vi "StepAmplitude.vi"() -> ()   [LabVIEW 2013]
uses:
  C:/Code/Apps/Utilities/AG-UC2-UC8/AG-UC2-UC8/Install/Samples/LabVIEW/LabVIEW 2013/CmdLibAgilis.dll
  CmdLibAgilis.dll
panel:
  out "Output:":string
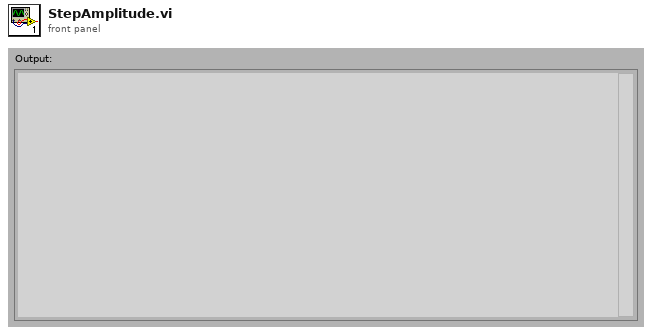
[diagram p1: front panel]
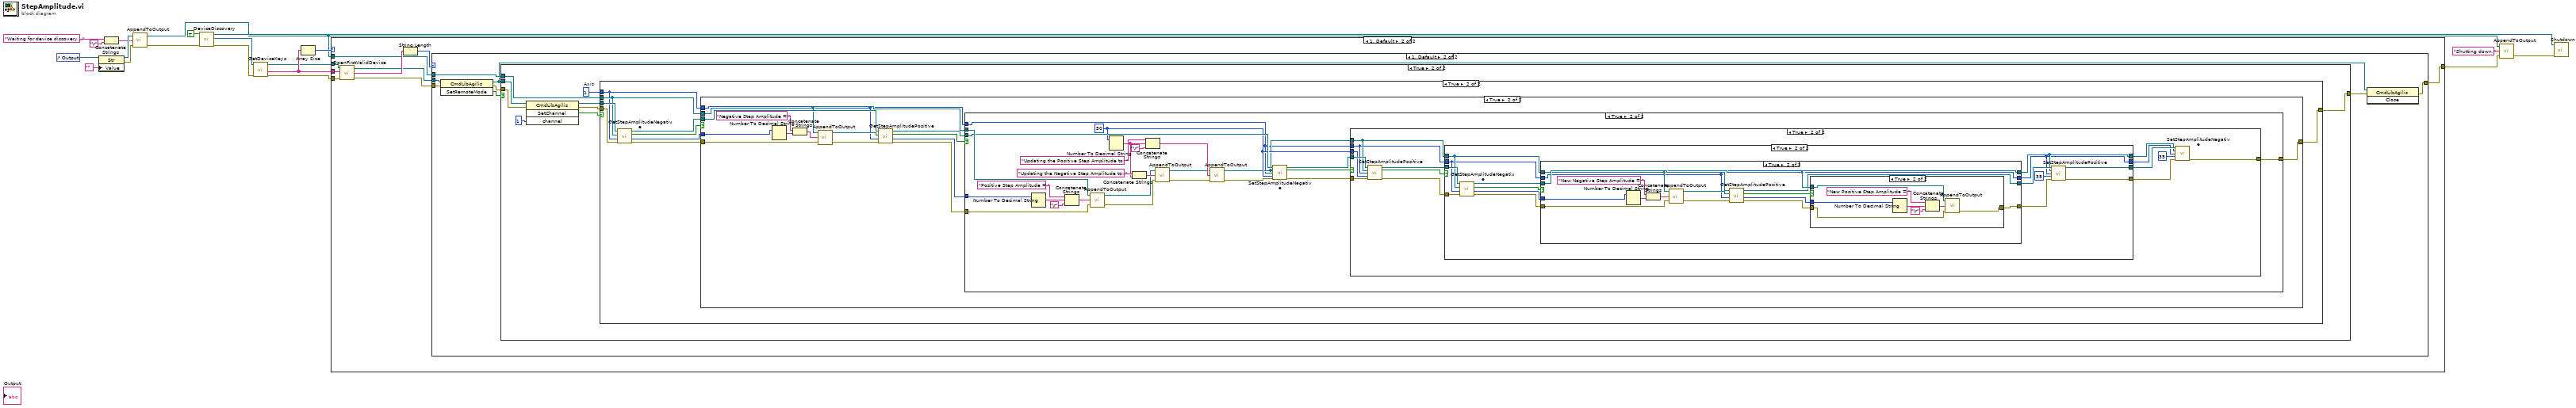
[diagram p0: block diagram]
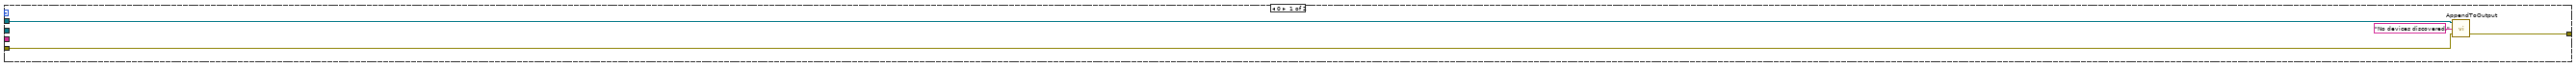
[diagram p2: hidden frame]
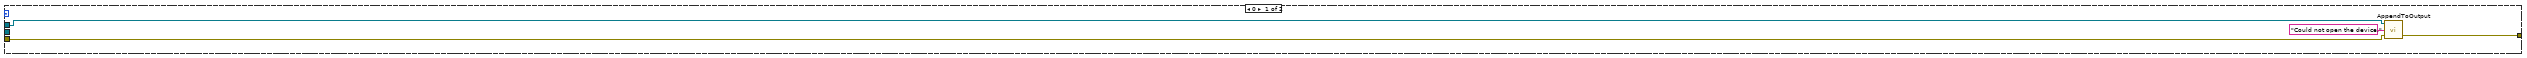
[diagram p3: hidden frame]
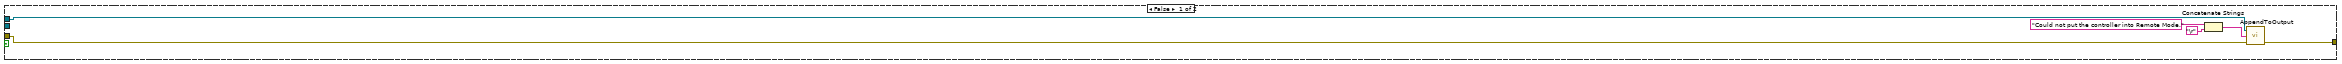
[diagram p4: hidden frame]
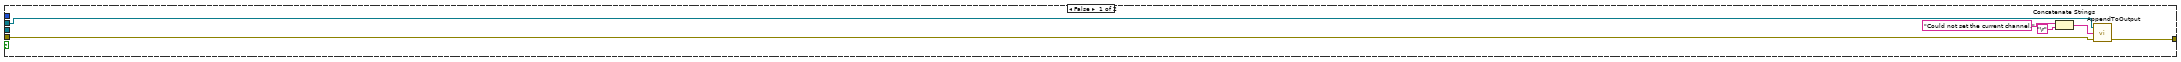
[diagram p5: hidden frame]
diagram:
  n1 = control-ref of="Output:"() -> (w20:refnum<vi>)
  n2 = property class="Str"(reference=w20, "Value"="") -> (reference out=w17:refnum<vi>, error out=w18:errorcluster)  [unwired: 1 in]
  n3 = Concatenate Strings("Waiting for device discovery...", "\r") -> (w7:string)
  n4 = call "AppendToOutput.vi"("error in"=w18, "Input String"=w7, "Output Refnum In"=w17) -> ("error out"=w15:errorcluster, "Output Refnum Out"=w1:refnum<vi>)  [unwired: 1 in]
  n5 = call "DeviceDiscovery.vi"("error in (no error)"=w15, "logging"=TRUE) -> ("error out"=w14:errorcluster, "CmdLib Out"=w13:refnum<k24>, "VCPIOLib Out"=w10:refnum<k24>)  [unwired: 3 in]
  n6 = call "GetDeviceKeys.vi"("error in (no error)"=w14, "CmdLib In"=w13) -> ("error out"=w11:errorcluster, "Device Keys"=w9:string[], "CmdLib Out"=w8:refnum<k24>)  [unwired: 3 in]
  n7 = Array Size(array=w9) -> (size(s)=w12:i32)
  n8 = case shown="1, Default" w12 {
    tunnel: w1 -> [w24 w28]
    tunnel: w11 -> [w23 w32]
    tunnel: w9 -> [_ w31]
    tunnel: w8 -> [_ w33]
    tunnel: [w21 w25] -> w2
    frame 0 {
      n9 = call "AppendToOutput.vi"("error in"=w23, "Input String"="No devices discovered.", "Output Refnum In"=w24) -> ("error out"=w21:errorcluster)  [unwired: 1 in, 1 out]
    }
    frame 1, Default {
      n10 = call "OpenFirstValidDevice.vi"("error in (no error)"=w32, "Device Keys"=w31, "CmdLib In"=w33) -> ("error out"=w27:errorcluster, "DeviceKey Out"=w30:string, "CmdLib Out"=w26:refnum<k24>)  [unwired: 1 in]
      n11 = String Length(string=w30) -> (length=w29:i32)
      n12 = case shown="1, Default" w29 {
        tunnel: w28 -> [w36 w42]
        tunnel: w27 -> [w35 w45]
        tunnel: w26 -> [_ w44]
        tunnel: [w34 w39] -> w25
        frame 0 {
          n13 = call "AppendToOutput.vi"("error in"=w35, "Input String"="Could not open the device." ("DeviceKey Out"), "Output Refnum In"=w36) -> ("error out"=w34:errorcluster)  [unwired: 1 in, 1 out]
        }
        frame 1, Default {
          n14 = invoke class="CmdLibAgilis" method="SetRemoteMode"(reference=w44, error in=w45) -> (reference out=w38:refnum<k24>, error out=w43:errorcluster, "SetRemoteMode"=w41:bool)  [unwired: 1 in]
          n15 = case shown="True" w41 {
            tunnel: w43 -> [w51 w60]
            tunnel: w42 -> [w47 w55]
            tunnel: w38 -> [_ w59]
            tunnel: [w46 w54] -> w40
            frame False {
              n16 = Concatenate Strings("Could not put the controller into Remote Mode." ("DeviceKey Out"), "\r") -> (w50:string)
              n17 = call "AppendToOutput.vi"("error in"=w51, "Input String"=w50, "Output Refnum In"=w47) -> ("error out"=w46:errorcluster)  [unwired: 1 in, 1 out]
            }
            frame True {
              w52 = 1  # Axis
              n18 = invoke class="CmdLibAgilis" method="SetChannel"(reference=w59, error in=w60, "channel"=1) -> (reference out=w53:refnum<k24>, error out=w56:errorcluster, "SetChannel"=w57:bool)  [unwired: 1 in, 1 out]
              n19 = case shown="True" w57 {
                tunnel: w55 -> [w66 w70]
                tunnel: w56 -> [w65 w74]
                tunnel: [w61 w71] -> w54
                tunnel: w53 -> [_ w75]
                tunnel: w52 -> [_ w68]
                frame False {
                  n20 = Concatenate Strings("Could not set the current channel." ("DeviceKey Out"), "\r") -> (w64:string)
                  n21 = call "AppendToOutput.vi"("error in"=w65, "Input String"=w64, "Output Refnum In"=w66) -> ("error out"=w61:errorcluster)  [unwired: 1 in, 1 out]
                }
                frame True {
                  n22 = call "GetStepAmplitudeNegative.vi"("error in (no error)"=w74, "Axis"=w68, "Output Refnum In"=w70, "CmdLib In"=w75) -> ("error out"=w69:errorcluster, "Step Amplitude"=w73:i32, "GetStepAmplitudeNegative"=w72:bool, "CmdLib Out"=w67:refnum<k24>)  [unwired: 4 in]
                  n23 = case shown="True" w72 {
                    tunnel: w73 -> [_ w90]
                    tunnel: [w76 w79] -> w71
                    tunnel: w70 -> [_ w80]
                    tunnel: w69 -> [w76 w87]
                    tunnel: w68 -> [_ w78]
                    tunnel: w67 -> [_ w84]
                    frame False {
                    }
                    frame True {
                      n24 = Number To Decimal String(number=w90) -> (decimal integer string=w89:string)  [unwired: 1 in]
                      n25 = Concatenate Strings("Negative Step Amplitude = ", w89) -> (w88:string)
                      n26 = call "AppendToOutput.vi"("error in"=w87, "Input String"=w88, "Output Refnum In"=w80) -> ("error out"=w86:errorcluster, "Output Refnum Out"=w85:refnum<vi>)  [unwired: 1 in]
                      n27 = call "GetStepAmplitudePositive.vi"("error in (no error)"=w86, "Axis"=w78, "Output Refnum In"=w85, "CmdLib In"=w84) -> ("error out"=w81:errorcluster, "Step Amplitude"=w82:i32, "GetStepAmplitudePositive"=w83:bool, "CmdLib Out"=w77:refnum<k24>)  [unwired: 4 in]
                      n28 = case shown="True" w83 {
                        tunnel: w82 -> [_ w115]
                        tunnel: w81 -> [w92 w114]
                        tunnel: w80 -> [_ w113]
                        tunnel: [w92 w93] -> w79
                        tunnel: w78 -> [_ w94]
                        tunnel: w77 -> [_ w100]
                        frame False {
                        }
                        frame True {
                          w96 = 50 ("Step Amplitude")
                          n29 = Number To Decimal String(number=w115) -> (decimal integer string=w117:string)  [unwired: 1 in]
                          n30 = Concatenate Strings("Positive Step Amplitude = ", w117, "\r") -> (w116:string)
                          n31 = call "AppendToOutput.vi"("error in"=w114, "Input String"=w116, "Output Refnum In"=w113) -> ("error out"=w111:errorcluster, "Output Refnum Out"=w103:refnum<vi>)  [unwired: 1 in]
                          n32 = Number To Decimal String(number=w96) -> (decimal integer string=w105:string)  [unwired: 1 in]
                          n33 = Concatenate Strings("Updating the Negative Step Amplitude to: " ("concatenated string"), w105) -> (w109:string)
                          n34 = Concatenate Strings("Updating the Positive Step Amplitude to: " ("concatenated string"), w105, "\r") -> (w108:string)
                          n35 = call "AppendToOutput.vi"("error in"=w111, "Input String"=w109, "Output Refnum In"=w103) -> ("error out"=w110:errorcluster, "Output Refnum Out"=w102:refnum<vi>)  [unwired: 1 in]
                          n36 = call "AppendToOutput.vi"("error in"=w110, "Input String"=w108, "Output Refnum In"=w102) -> ("error out"=w101:errorcluster, "Output Refnum Out"=w95:refnum<vi>)  [unwired: 1 in]
                          n37 = call "SetStepAmplitudeNegative.vi"("CmdLib In"=w100, "Output Refnum In"=w95, "Axis"=w94, "Step Amplitude"=w96, "error in (no error)"=w101) -> ("CmdLib Out"=w97:refnum<k24>, "SetStepAmplitudeNegative"=w99:bool, "error out"=w98:errorcluster)  [unwired: 8 in]
                          n38 = case shown="True" w99 {
                            tunnel: w98 -> [w119 w132]
                            tunnel: w97 -> [_ w133]
                            tunnel: w96 -> [_ w131]
                            tunnel: w95 -> [_ w126]
                            tunnel: w94 -> [_ w127]
                            tunnel: [w119 w120] -> w93
                            frame False {
                            }
                            frame True {
                              n39 = call "SetStepAmplitudePositive.vi"("CmdLib In"=w133, "Output Refnum In"=w126, "Axis"=w127, "Step Amplitude"=w131, "error in (no error)"=w132) -> ("CmdLib Out"=w129:refnum<k24>, "SetStepAmplitudePositive"=w130:bool, "error out"=w128:errorcluster)  [unwired: 8 in]
                              n40 = case shown="True" w130 {
                                tunnel: w129 -> [w136 w152]
                                tunnel: w128 -> [w134 w151]
                                tunnel: w127 -> [w135 w145]
                                tunnel: w126 -> [w137 w148]
                                tunnel: [w136 w141] -> w125
                                tunnel: [w134 w140] -> w124
                                tunnel: [w137 w139] -> w123
                                tunnel: [w135 w138] -> w122
                                frame False {
                                }
                                frame True {
                                n41 = call "GetStepAmplitudeNegative.vi"("error in (no error)"=w151, "Axis"=w145, "Output Refnum In"=w148, "CmdLib In"=w152) -> ("error out"=w149:errorcluster, "Step Amplitude"=w147:i32, "GetStepAmplitudeNegative"=w150:bool, "CmdLib Out"=w146:refnum<k24>)  [unwired: 4 in]
                                n42 = case shown="True" w150 {
                                tunnel: w149 -> [w153 w170]
                                tunnel: w148 -> [w155 w160]
                                tunnel: w147 -> [_ w167]
                                tunnel: w146 -> [w154 w164]
                                tunnel: w145 -> [w156 w158]
                                tunnel: [w156 w158] -> w138
                                tunnel: [w155 w160] -> w139
                                tunnel: [w154 w159] -> w144
                                tunnel: [w153 w161] -> w143
                                frame False {
                                }
                                frame True {
                                n43 = Number To Decimal String(number=w167) -> (decimal integer string=w169:string)  [unwired: 1 in]
                                n44 = Concatenate Strings("New Negative Step Amplitude = ", w169) -> (w168:string)
                                n45 = call "AppendToOutput.vi"("error in"=w170, "Input String"=w168, "Output Refnum In"=w160) -> ("error out"=w165:errorcluster, "Output Refnum Out"=w166:refnum<vi>)  [unwired: 1 in]
                                n46 = call "GetStepAmplitudePositive.vi"("error in (no error)"=w165, "Axis"=w158, "Output Refnum In"=w166, "CmdLib In"=w164) -> ("error out"=w162:errorcluster, "Step Amplitude"=w157:i32, "GetStepAmplitudePositive"=w163:bool, "CmdLib Out"=w159:refnum<k24>)  [unwired: 4 in]
                                n47 = case shown="True" w163 {
                                tunnel: w160 -> [_ w177]
                                tunnel: w162 -> [w172 w176]
                                tunnel: [w172 w174] -> w161
                                tunnel: w157 -> [_ w173]
                                frame False {
                                }
                                frame True {
                                n48 = Number To Decimal String(number=w173) -> (decimal integer string=w179:string)  [unwired: 1 in]
                                n49 = Concatenate Strings("New Positive Step Amplitude = ", w179, "\r") -> (w178:string)
                                n50 = call "AppendToOutput.vi"("error in"=w176, "Input String"=w178, "Output Refnum In"=w177) -> ("error out"=w174:errorcluster)  [unwired: 1 in, 1 out]
                                }
                                }
                                }
                                }
                                n51 = call "SetStepAmplitudePositive.vi"("CmdLib In"=w144, "Output Refnum In"=w139, "Axis"=w138, "Step Amplitude"=35, "error in (no error)"=w143) -> ("CmdLib Out"=w141:refnum<k24>, "error out"=w140:errorcluster)  [unwired: 8 in, 1 out]
                                }
                              }
                              n52 = call "SetStepAmplitudeNegative.vi"("CmdLib In"=w125, "Output Refnum In"=w123, "Axis"=w122, "Step Amplitude"=35, "error in (no error)"=w124) -> ("error out"=w120:errorcluster)  [unwired: 8 in, 2 out]
                            }
                          }
                        }
                      }
                    }
                  }
                }
              }
            }
          }
          n53 = invoke class="CmdLibAgilis" method="Close"(reference=w38, error in=w40) -> (error out=w39:errorcluster)  [unwired: 1 in, 2 out]
        }
      }
    }
  }
  n54 = call "AppendToOutput.vi"("error in"=w2, "Input String"="Shutting down." ("concatenated string"), "Output Refnum In"=w1) -> ("error out"=w3:errorcluster)  [unwired: 1 in, 1 out]
  n55 = call "Shutdown.vi"("error in (no error)"=w3, "VCPIOLib In"=w10) -> ()  [unwired: 9 in, 1 out]
